vi "checkHostFree.vi"(0 "Host_Reference":refnum<class "HGF_Reference.lvclass">, 2 "timeout in ms (-1)":i32, 5 "error in (no error)":errorcluster) -> (14 "dup Host_Reference":refnum<class "HGF_Reference.lvclass">, 16 "dup timeout in ms (-1)":i32, 17 "free4agents":bool=TRUE, 19 "error out":errorcluster)   [LabVIEW 2009, in "MoAgSy.lvlib" / "MoAgSy_Host.lvclass"]
doc: "<B>public</B> VI checks if number of running Agents is less than max number of Agents of referenced Host.\n\nF.Berck@gsi.de\nGSI Darmstadt 2009"
uses:
  MoAgSy_Host.lvclass
  HGF_BaseClasses/HGF_Reference/HGF_Reference.lvclass
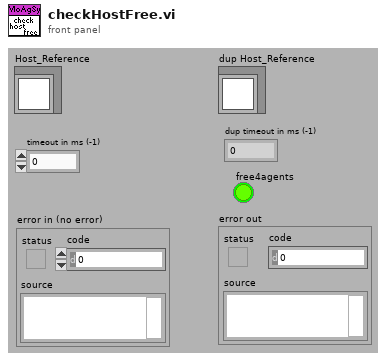
[diagram p1: front panel]
types:
  T1 = cluster{"Host Name":string, "Maximum number of running Agents":i16, "ID":string}
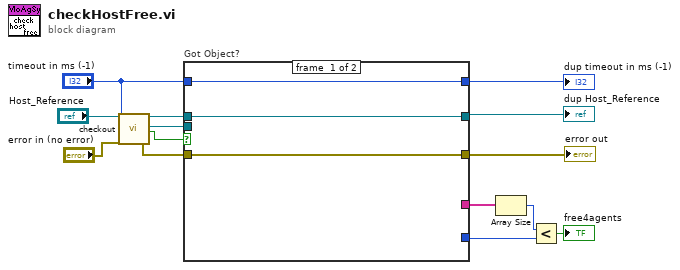
[diagram p0: block diagram]
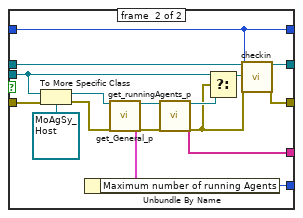
[diagram p2: hidden frame]
diagram:
  n1 = call "checkout.vi"("HGF_Reference"="Host_Reference", "timeout in ms (-1)"="timeout in ms (-1)", "error in (no error)"="error in (no error)") -> ("dup HGF_Reference"=w14:refnum<class "HGF_Reference.lvclass">, "Object"=w12:refnum<class>, "got object?"=w13:bool, "error out"=w11:errorcluster)  [unwired: 13 out]
  n2 = case "Got Object?" shown="True" w13 {
    tunnel: w11 -> [w16 w34]
    tunnel: w12 -> [_ w29]
    tunnel: w14 -> [w17 w32]
    tunnel: [w17 w31] -> w8
    tunnel: "timeout in ms (-1)" -> [w15 w27]
    tunnel: [w16 w30] -> w5
    tunnel: [w15 w27] -> w6
    tunnel: [_ w23] -> w2
    tunnel: [_ w19] -> w4
    frame #0 {
    }
    frame #1 {
      n3 = To More Specific Class(target class=refnum<class "MoAgSy_Host.lvclass"> refnum ("MoAgSy.lvlib:MoAgSy_Host.lvclass"), reference=w29, error in=w34) -> (specific class reference=w26:refnum<class "MoAgSy_Host.lvclass">, error out=w25:errorcluster)
      n4 = call "get_General_p.vi"("MoAgSy_Host"=w26, "error in (no error)"=w25) -> ("dup MoAgSy_Host"=w22:refnum<class "MoAgSy_Host.lvclass">, "General"=w24:T1, "error out"=w21:errorcluster)  [unwired: 15 out]
      n5 = Unbundle By Name(w24) -> ("Maximum number of running Agents"=w23:i16)
      n6 = call "get_runningAgents_p.vi"("MoAgSy_Host"=w22, "error in (no error)"=w21) -> ("dup MoAgSy_Host"=w20:refnum<class "MoAgSy_Host.lvclass">, "Running Agents"=w19:string[], "error out"=w18:errorcluster)  [unwired: 15 out]
      n7 = Select(t=w29, s=w18, f=w20) -> (s? t:f=w28:refnum<class>)
      n8 = call "checkin.vi"("HGF_Reference"=w32, "Object"=w28, "timeout /ms (-1)"=w27, "error in (no error)"=w18) -> ("dup HGF_Reference"=w31:refnum<class "HGF_Reference.lvclass">, "error out"=w30:errorcluster)  [unwired: 14 out]
    }
  }
  "dup Host_Reference" <- w8
  "dup timeout in ms (-1)" <- w6
  "error out" <- w5
  n9 = Array Size(array=w4) -> (size(s)=w3:i32)
  n10 = Less?(x=w3, y=w2) -> (x < y?=→"free4agents":bool)
